vi "initial.vi"() -> ()   [LabVIEW 2022 SP3]
uses:
  <vilib>/DAQmx/read.llb/DAQmx Read (Analog DBL 1Chan 1Samp).vi
  <vilib>/DAQmx/write.llb/DAQmx Write (Digital Bool 1Line 1Point).vi
  <vilib>/DAQmx/create/channels.llb/DAQmx Create Channel (DO-Digital Output).vi
  <vilib>/DAQmx/miscellaneous.llb/DAQmx Fill In Error Info.vi
  <vilib>/DAQmx/create/channels.llb/DAQmx Create Channel (AI-Voltage-Basic).vi
  Reading Blue.vi
  Reading Green.vi
  Reading Red.vi
panel:
  out "Array":dbl[](array[numeric])
  out "Numeric 2":i32
  out "red":bool
  out "blue":bool
  out "green":bool
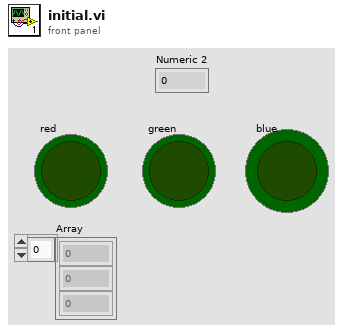
[diagram p1: front panel]
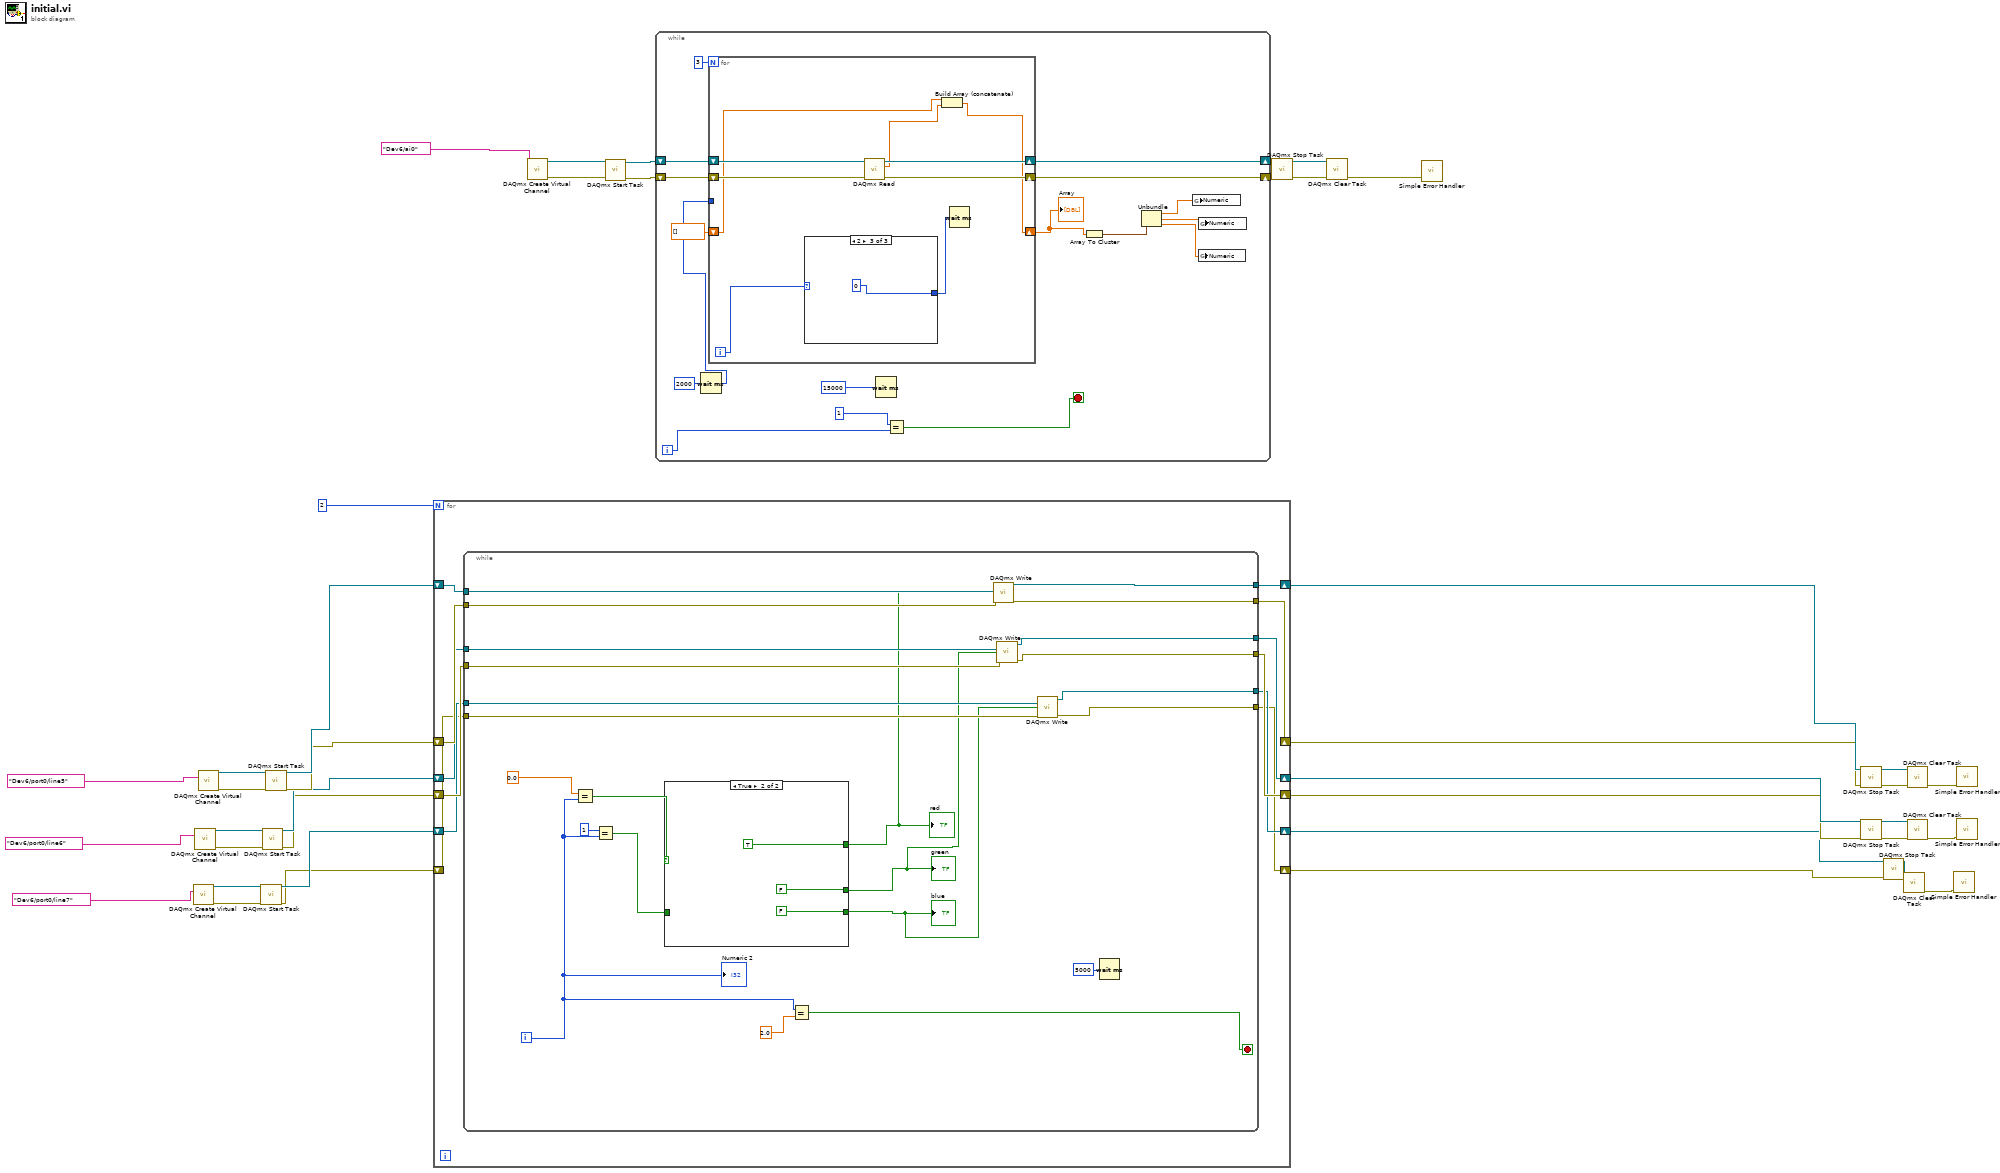
[diagram p0: block diagram]
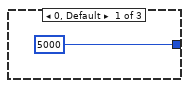
[diagram p2: hidden frame]
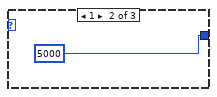
[diagram p3: hidden frame]
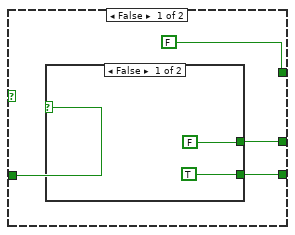
[diagram p4: hidden frame]
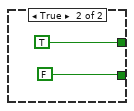
[diagram p5: hidden frame]
diagram:
  n1 = call-poly <vilib>:"DAQmx Create Virtual Channel.vi"("lines"=tag "Dev6/port0/line7" ("Blue Channel")) -> ("task out"=w30:refnum<k21>, "error out"=w31:errorcluster)  [unwired: 13 in]
  n2 = call-poly <vilib>:"DAQmx Create Virtual Channel.vi"("lines"=tag "Dev6/port0/line6" ("Green Channel")) -> ("task out"=w35:refnum<k21>, "error out"=w36:errorcluster)  [unwired: 13 in]
  n3 = call-poly <vilib>:"DAQmx Create Virtual Channel.vi"("lines"=tag "Dev6/port0/line5" ("Red Channel")) -> ("task out"=w40:refnum<k21>, "error out"=w41:errorcluster)  [unwired: 13 in]
  n4 = call <vilib>:"DAQmx Start Task.vi"("task/channels in"=w30, "error in"=w31) -> ("task out"=w19:refnum<k21>, "error out"=w18:errorcluster)  [unwired: 12 in]
  n5 = call <vilib>:"DAQmx Start Task.vi"("task/channels in"=w35, "error in"=w36) -> ("task out"=w21:refnum<k21>, "error out"=w20:errorcluster)  [unwired: 12 in]
  n6 = call <vilib>:"DAQmx Start Task.vi"("task/channels in"=w40, "error in"=w41) -> ("task out"=w23:refnum<k21>, "error out"=w22:errorcluster)  [unwired: 12 in]
  n7 = for {
    N: 2 -> [_]
    shift-right: [w47] -> w17
    shift-left: w23 -> [w53]
    shift-right: [w46] -> w16
    shift-left: w22 -> [w52]
    shift-right: [w45] -> w15
    shift-left: w21 -> [w51]
    shift-right: [w44] -> w14
    shift-left: w20 -> [w50]
    shift-right: [w43] -> w13
    shift-left: w19 -> [w49]
    shift-right: [w42] -> w12
    shift-left: w18 -> [w48]
    n8 = while {
      tunnel: w53 -> [w68]
      tunnel: w52 -> [w67]
      tunnel: [w66] -> w47
      tunnel: [w65] -> w46
      tunnel: w51 -> [w64]
      tunnel: w50 -> [w63]
      tunnel: [w62] -> w45
      tunnel: [w61] -> w44
      tunnel: w49 -> [w60]
      tunnel: w48 -> [w59]
      tunnel: [w58] -> w43
      tunnel: [w57] -> w42
      i -> [w70]
      stop <- w75 stop-if-true
      n9 = Equal?(x=0.0, y=w70) -> (x = y?=w72:bool)
      n10 = Equal?(x=1, y=w70) -> (x = y?=w71:bool)
      n11 = case shown="True" w72 {
        tunnel: [FALSE TRUE] -> w56
        tunnel: w71 -> [w80 _]
        tunnel: [w78 FALSE] -> w54
        tunnel: [w77 FALSE] -> w55
        frame False {
          n12 = case shown="False" w80 {
            tunnel: [FALSE TRUE] -> w78
            tunnel: [TRUE FALSE] -> w77
            frame False {
            }
            frame True {
            }
          }
        }
        frame True {
        }
      }
      "red" <- w56
      "blue" <- w55
      "green" <- w54
      n13 = Equal?(x=w70, y=2.0) -> (x = y?=w75:bool)
      n14 = call-poly <vilib>:"DAQmx Write.vi"("task/channels in"=w68, "data"=w56, "error in"=w67) -> ("task out"=w66:refnum<k21>, "error out"=w65:errorcluster)  [unwired: 10 in, 1 out]
      n15 = call-poly <vilib>:"DAQmx Write.vi"("task/channels in"=w64, "data"=w54, "error in"=w63) -> ("task out"=w62:refnum<k21>, "error out"=w61:errorcluster)  [unwired: 10 in, 1 out]
      n16 = call-poly <vilib>:"DAQmx Write.vi"("task/channels in"=w60, "data"=w55, "error in"=w59) -> ("task out"=w58:refnum<k21>, "error out"=w57:errorcluster)  [unwired: 10 in, 1 out]
      n17 = Wait (ms)(milliseconds to wait=u32 5000) -> ()  [unwired: 1 out]
      "Numeric 2" <- w70
    }
  }
  n18 = call-poly <vilib>:"DAQmx Create Virtual Channel.vi"("physical channels"=tag "Dev6/ai0") -> ("task out"=w9:refnum<k21>, "error out"=w10:errorcluster)  [unwired: 13 in]
  n19 = call <vilib>:"DAQmx Start Task.vi"("task/channels in"=w9, "error in"=w10) -> ("task out"=w5:refnum<k21>, "error out"=w4:errorcluster)  [unwired: 12 in]
  n20 = while {
    shift-right: [w102] -> w3
    shift-left: w5 -> [w104]
    shift-right: [w101] -> w2
    shift-left: w4 -> [w103]
    i -> [w90]
    stop <- w88 stop-if-true
    n21 = Wait (ms)(milliseconds to wait=u32 2000) -> (millisecond timer value=w97:u32)
    n22 = for {
      N: 3 -> [_]
      shift-right: [w111] -> w102
      shift-left: w104 -> [w113]
      shift-right: [w110] -> w101
      shift-left: w103 -> [w112]
      shift-right: [w106] -> w95
      shift-left: dbl[] [] -> [w108]
      tunnel: w97 -> [_]
      i -> [w109]
      n23 = case shown="2" w109 {
        tunnel: [u32 5000 ("milliseconds to wait") u32 5000 ("milliseconds to wait") u32 0 ("milliseconds to wait")] -> w105
        frame 0, Default {
        }
        frame 1 {
        }
        frame 2 {
        }
      }
      n24 = call-poly <vilib>:"DAQmx Read.vi"("task/channels in"=w113, "error in"=w112) -> ("task out"=w111:refnum<k21>, "data"=w107:dbl, "error out"=w110:errorcluster)  [unwired: 11 in]
      n25 = Build Array (concatenate)(w108, w107) -> (w106:dbl[])
      n26 = Wait (ms)(milliseconds to wait=w105) -> ()  [unwired: 1 out]
    }
    "Array" <- w95
    n27 = Wait (ms)(milliseconds to wait=u32 15000 ("millisecond timer value")) -> ()  [unwired: 1 out]
    n28 = Equal?(x=1, y=w90) -> (x = y?=w88:bool)
    n29 = Array To Cluster(array=w95) -> (cluster=w94:cluster{"[0]":dbl, "[1]":dbl, "[2]":dbl})
    n30 = Unbundle "Unbundle"(w94) -> ("[0]"=w93:dbl, "[1]"=w92:dbl, "[2]"=w91:dbl)
    n31 = global write "Reading Red.vi" "Numeric"(w93) -> ()
    n32 = global write "Reading Blue.vi" "Numeric"(w91) -> ()
    n33 = global write "Reading Green.vi" "Numeric"(w92) -> ()
  }
  n34 = call <vilib>:"DAQmx Stop Task.vi"("task/channels in"=w3, "error in"=w2) -> ("task out"=w8:refnum<k21>, "error out"=w7:errorcluster)  [unwired: 12 in]
  n35 = call <vilib>:"DAQmx Clear Task.vi"("task in"=w8, "error in"=w7) -> ("error out"=w6:errorcluster)  [unwired: 13 in]
  n36 = call <vilib>:"Simple Error Handler.vi"("error in (no error)"=w6) -> ()  [unwired: 4 in, 5 out]
  n37 = call <vilib>:"DAQmx Stop Task.vi"("task/channels in"=w17, "error in"=w16) -> ("task out"=w39:refnum<k21>, "error out"=w38:errorcluster)  [unwired: 12 in]
  n38 = call <vilib>:"DAQmx Stop Task.vi"("task/channels in"=w15, "error in"=w14) -> ("task out"=w34:refnum<k21>, "error out"=w33:errorcluster)  [unwired: 12 in]
  n39 = call <vilib>:"DAQmx Stop Task.vi"("task/channels in"=w13, "error in"=w12) -> ("task out"=w29:refnum<k21>, "error out"=w28:errorcluster)  [unwired: 12 in]
  n40 = call <vilib>:"DAQmx Clear Task.vi"("task in"=w29, "error in"=w28) -> ("error out"=w27:errorcluster)  [unwired: 13 in]
  n41 = call <vilib>:"DAQmx Clear Task.vi"("task in"=w39, "error in"=w38) -> ("error out"=w37:errorcluster)  [unwired: 13 in]
  n42 = call <vilib>:"DAQmx Clear Task.vi"("task in"=w34, "error in"=w33) -> ("error out"=w32:errorcluster)  [unwired: 13 in]
  n43 = call <vilib>:"Simple Error Handler.vi"("error in (no error)"=w27) -> ()  [unwired: 4 in, 5 out]
  n44 = call <vilib>:"Simple Error Handler.vi"("error in (no error)"=w37) -> ()  [unwired: 4 in, 5 out]
  n45 = call <vilib>:"Simple Error Handler.vi"("error in (no error)"=w32) -> ()  [unwired: 4 in, 5 out]
